vi "GV-YscaleDetectArea.vi"(6 "GraphCursorLoc":T1, 8 "error in (no error)":errorcluster, 9 "X-position":i16, 10 "Plot":i32, 11 "Gviewer in":refnum<class "Gviewer.lvclass">) -> (0 "error out":errorcluster, 3 "Gviewer out":refnum<class "Gviewer.lvclass">)   [LabVIEW 2020, in "Sgraph_lib_V1.lvlib" / "Gviewer.lvclass"]
doc: "Draw an Y-scale on the graph canvas"
uses:
  Gviewer.lvclass
  <vilib>/Utility/miscctls.llb/LVPoint32TypeDef.ctl
  Gviewer.lvclass/Gviewer.ctl
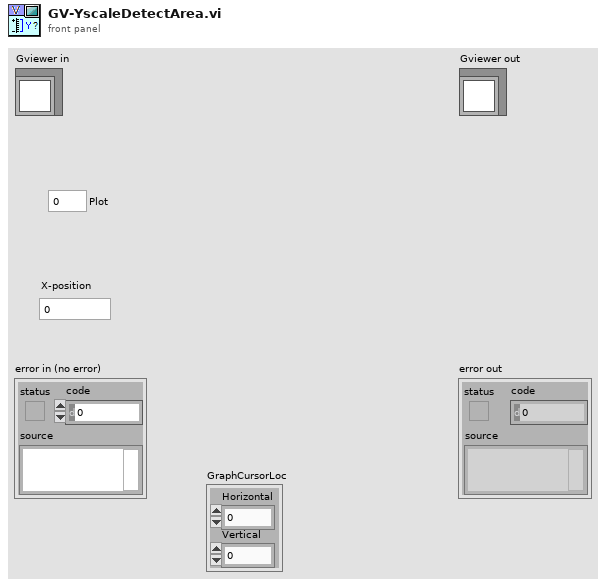
[diagram p1: front panel]
types:
  T1 = typedef "LVPoint32TypeDef.ctl" = cluster{"Horizontal":i32, "Vertical":i32}
  T2 = cluster{"data":dbl[], "max":dbl[], "min":dbl[], "Status":u32[]}[]
  T3 = typedef "Sgraph_lib_V1.lvlib/Gviewer.lvclass/Typedef_SelProperties.ctl" = cluster{"Color":u32, "LineType":T4, "max":dbl, "min":dbl, "unit":string}
  T4 = typedef "Sgraph_lib_V1.lvlib/Gviewer.lvclass/Typedef_LineType.ctl" = enum16{"num_bare", "num_MinMax_Area", "num_MinMax_Lines", "num_MinMax_Forfor", "num_Max_Area", "num_Max_Line", "num_Max_Forfor", "num_Min_Area", "num_Min_Line", "num_Min_Fosfor", "Boolean_Line_01", "Boolean_Area_01", "Boolean_Fosfor_01", "Boolean_Line_TF", "Boolean_Area_TF", "Boolean_Fosfor_TF", "Boolean_OnOff_Line", "Boolean_OnOff_Area", "Boolean_OnOff_Fosfor", "Boolean_spare", "StringEvent_Line", "StringEvent_TimeLine"}
  T5 = cluster{"data":dbl[], "max":dbl[], "min":dbl[], "Status":u32[]}
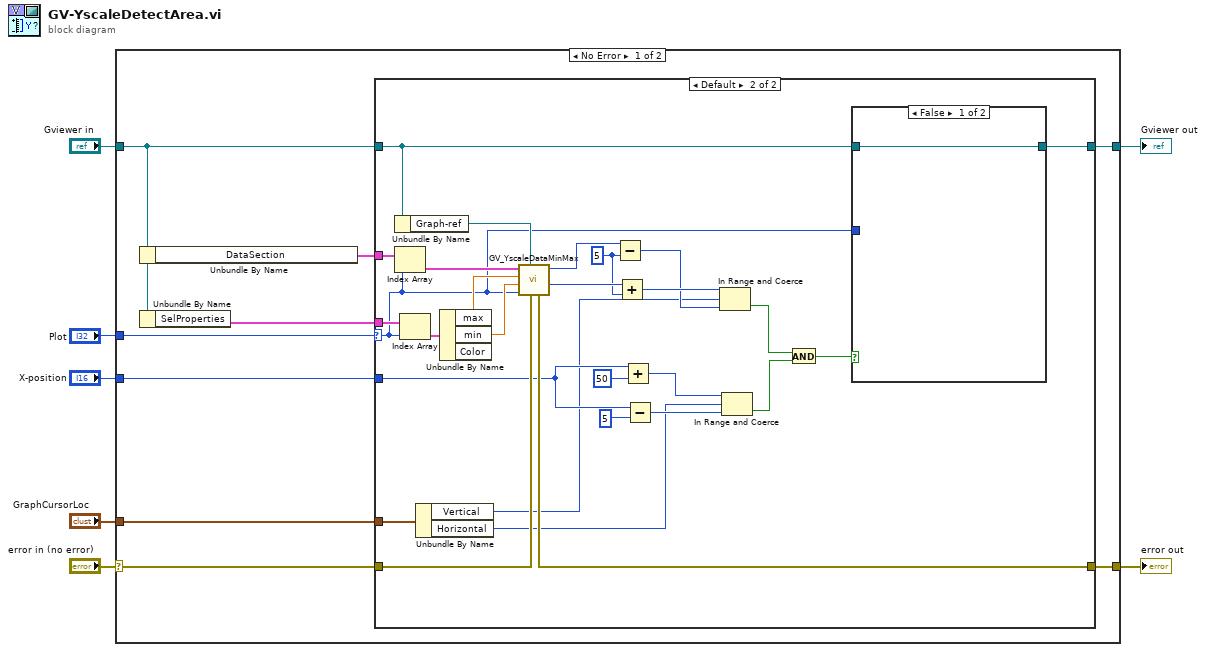
[diagram p0: block diagram]
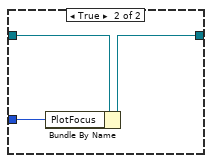
[diagram p3: hidden frame]
diagram:
  n1 = case shown="No Error" "error in (no error)" {
    selector: "error in (no error)" -> [w11 w52]
    tunnel: [w10 w52] -> w6
    tunnel: [w9 w51] -> w4
    tunnel: "Gviewer in" -> [w13 w51]
    tunnel: "X-position" -> [w16 _]
    tunnel: "Plot" -> [w12 _]
    tunnel: "GraphCursorLoc" -> [w8 _]
    frame No Error {
      n2 = Unbundle By Name(w13) -> ("DataSection"=w14:T2)
      n3 = Unbundle By Name(w13) -> ("SelProperties"=w15:T3[])
      n4 = case shown="Default" w12 {
        selector: w12 -> [_ w19]
        tunnel: w16 -> [_ w31]
        tunnel: w15 -> [_ w46]
        tunnel: w14 -> [_ w44]
        tunnel: w13 -> [w18 w21]
        tunnel: w11 -> [w17 w41]
        tunnel: [w17 w38] -> w10
        tunnel: [w18 w20] -> w9
        tunnel: w8 -> [_ w28]
        frame -1 {
        }
        frame Default {
          w35 = 5 ("y")
          n5 = Unbundle By Name(w21) -> ("Graph-ref"=w42:refnum<vi>)
          n6 = Index Array(array=w44, index=w19) -> (element=w43:T5)
          n7 = Index Array(array=w46, index=w19) -> (element=w45:T3)
          n8 = Unbundle By Name(w28) -> ("Vertical"=w27:i32, "Horizontal"=w26:i32)
          n9 = Unbundle By Name(w45) -> ("max"=w40:dbl, "min"=w39:dbl)  [unwired: 1 out]
          n10 = call "GV_YscaleDataMinMax.vi"("error in (no error)"=w41, "Graph-ref"=w42, "Plot"=w19, "Scale-min"=w39, "Scale-max"=w40, "PAQ-data"=w43) -> ("Coord-min"=w36:i32, "Coord-max"=w37:i32, "error out"=w38:errorcluster)  [unwired: 1 in, 2 out]
          n11 = Subtract(x=w37, y=w35) -> (x-y=w33:i32)
          n12 = Add(x=w36, y=w35) -> (x+y=w34:i32)
          n13 = Add(x=w31, y=50) -> (x+y=w30:i32)
          n14 = Subtract(x=w31, y=5) -> (x-y=w29:i32)
          n15 = In Range and Coerce(upper limit=w34, x=w27, lower limit=w33) -> (In Range?=w25:bool)  [unwired: 1 out]
          n16 = In Range and Coerce(upper limit=w30, x=w26, lower limit=w29) -> (In Range?=w24:bool)  [unwired: 1 out]
          n17 = And(x=w25, y=w24) -> (x .and. y?=w22:bool)
          n18 = case shown="False" w22 {
            tunnel: w21 -> [w47 w50]
            tunnel: [w47 w48] -> w20
            tunnel: w19 -> [_ w49]
            frame False {
            }
            frame True {
              n19 = Bundle By Name(cluster=w50, "PlotFocus"=w49) -> (w48:refnum<class "Gviewer.lvclass">)
            }
          }
        }
      }
    }
    frame Error {
    }
  }
  "error out" <- w6
  "Gviewer out" <- w4
